vi "Node Status to gRPC Status.vi"(2 "Node Status":T1 {"Custom 8" format="%#_13g"}) -> (4 "gRPC Status":T4)   [LabVIEW 2021, in "CIFTemplateCommon.lvlib"]
uses:
  CIFTemplateCommon.lvlib
  CIFNodeCoreGrpc/CIFNodeCoreGrpc_server/RPC Messages/cif_nodecore_StatusData.ctl
  CIFNodeCoreGrpc/CIFNodeCoreGrpc_server/RPC Messages/cif_nodecore_StatusData_State.ctl
  CIFNodeCoreGrpc/CIFNodeCoreGrpc_server/RPC Messages/cif_nodecore_Error.ctl
  Typedef/Plugin Status.ctl
  Typedef/Plugin State.ctl
  Typedef/Simple Error.ctl
  CIFNodeCoreGrpc/CIFNodeCoreGrpc_server/CIFNodeCoreGrpc_server.lvlib
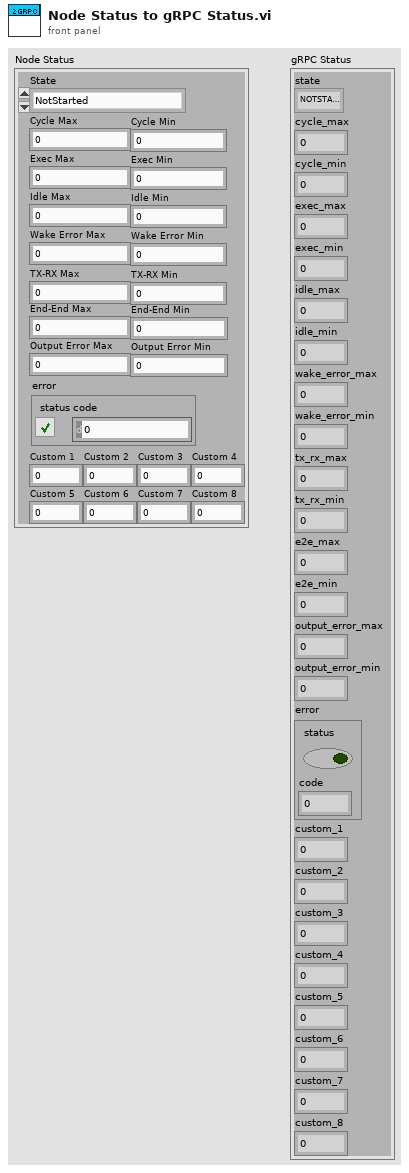
[diagram p1: front panel]
types:
  T1 = typedef "CIFTemplateCommon.lvlib/Plugin Status.ctl" = cluster{"State":T2, "Cycle Max":i32, "Cycle Min":i32, "Exec Max":i32, "Exec Min":i32, "Idle Max":i32, "Idle Min":i32, "Wake Error Max":i32, "Wake Error Min":i32, "TX-RX Max":i32, "TX-RX Min":i32, "End-End Max":i32, "End-End Min":i32, "Output Error Max":i32, "Output Error Min":i32, "error":T3, "Custom 1":u64, "Custom 2":u64, "Custom 3":u64, "Custom 4":u64, "Custom 5":dbl, "Custom 6":dbl, "Custom 7":dbl, "Custom 8":dbl}
  T2 = typedef "CIFTemplateCommon.lvlib/Plugin State.ctl" = enum32{"NotStarted", "Initialized", "Ready", "Running", "Shutdown"}
  T3 = typedef "CIFTemplateCommon.lvlib/Simple Error.ctl" = cluster{"status":bool, "code":i32}
  T4 = typedef "CIFNodeCoreGrpc_server.lvlib/cif_nodecore_StatusData.ctl" = cluster{"state":T5, "cycle_max":i32, "cycle_min":i32, "exec_max":i32, "exec_min":i32, "idle_max":i32, "idle_min":i32, "wake_error_max":i32, "wake_error_min":i32, "tx_rx_max":i32, "tx_rx_min":i32, "e2e_max":i32, "e2e_min":i32, "output_error_max":i32, "output_error_min":i32, "error":T6, "custom_1":u64, "custom_2":u64, "custom_3":u64, "custom_4":u64, "custom_5":dbl, "custom_6":dbl, "custom_7":dbl, "custom_8":dbl}
  T5 = typedef "CIFNodeCoreGrpc_server.lvlib/cif_nodecore_StatusData_State.ctl" = enum32{"NOTSTARTED", "INITIALIZED", "READY", "RUNNING", "SHUTDOWN"}
  T6 = typedef "CIFNodeCoreGrpc_server.lvlib/cif_nodecore_Error.ctl" = cluster{"status":bool, "code":i32}
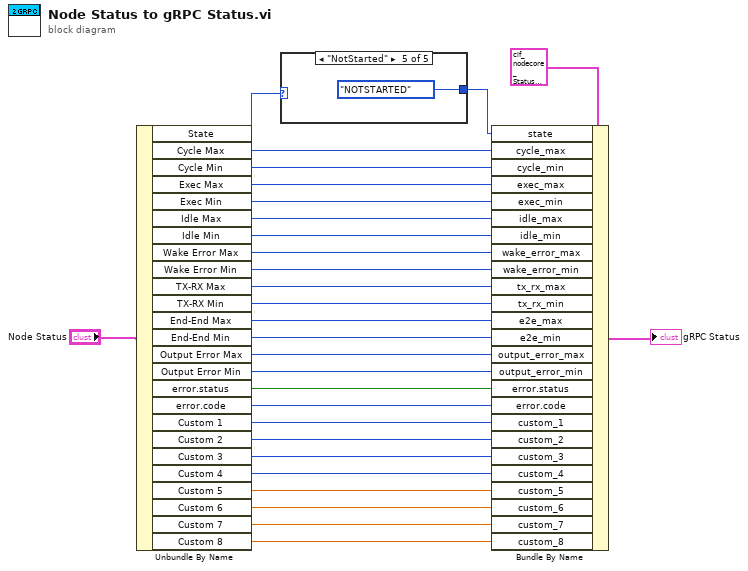
[diagram p0: block diagram]
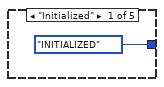
[diagram p2: hidden frame]
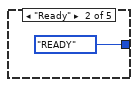
[diagram p3: hidden frame]
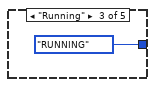
[diagram p4: hidden frame]
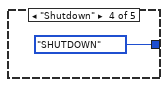
[diagram p5: hidden frame]
diagram:
  n1 = Unbundle By Name("Node Status") -> ("State"=w25:T2, "Cycle Max"=w24:i32, "Cycle Min"=w23:i32, "Exec Max"=w22:i32, "Exec Min"=w21:i32, "Idle Max"=w20:i32, "Idle Min"=w19:i32, "Wake Error Max"=w18:i32, "Wake Error Min"=w17:i32, "TX-RX Max"=w16:i32, "TX-RX Min"=w15:i32, "End-End Max"=w14:i32, "End-End Min"=w13:i32, "Output Error Max"=w12:i32, "Output Error Min"=w11:i32, "error.status"=w10:bool, "error.code"=w9:i32, "Custom 1"=w1:u64, "Custom 2"=w2:u64, "Custom 3"=w3:u64, "Custom 4"=w4:u64, "Custom 5"=w5:dbl, "Custom 6"=w6:dbl, "Custom 7"=w7:dbl, "Custom 8"=w8:dbl)
  n2 = case shown="\"NotStarted\"" w25 {
    tunnel: [cif_nodecore_StatusData_State."INITIALIZED" ("state") cif_nodecore_StatusData_State."READY" ("state") cif_nodecore_StatusData_State."RUNNING" ("state") cif_nodecore_StatusData_State."SHUTDOWN" ("state") cif_nodecore_StatusData_State."NOTSTARTED" ("state")] -> w26
    frame "Initialized" {
    }
    frame "Ready" {
    }
    frame "Running" {
    }
    frame "Shutdown" {
    }
    frame "NotStarted" {
    }
  }
  n3 = Bundle By Name(cluster=T4 {"state"=enum."NOTSTARTED", "cycle_max"=0, "cycle_min"=0, "exec_max"=0, "exec_min"=0, "idle_max"=0, "idle_min"=0, "wake_error_max"=0, "wake_error_min"=0, "tx_rx_max"=0, "tx_rx_min"=0, "e2e_max"=0, "e2e_min"=0, "output_error_max"=0, "output_error_min"=0, "error"={"status"=FALSE, "code"=0}, "custom_1"=0, "custom_2"=0, "custom_3"=0, "custom_4"=0, "custom_5"=0.0, "custom_6"=0.0, "custom_7"=0.0, "custom_8"=0.0} ("Message Data"), "state"=w26, "cycle_max"=w24, "cycle_min"=w23, "exec_max"=w22, "exec_min"=w21, "idle_max"=w20, "idle_min"=w19, "wake_error_max"=w18, "wake_error_min"=w17, "tx_rx_max"=w16, "tx_rx_min"=w15, "e2e_max"=w14, "e2e_min"=w13, "output_error_max"=w12, "output_error_min"=w11, "error.status"=w10, "error.code"=w9, "custom_1"=w1, "custom_2"=w2, "custom_3"=w3, "custom_4"=w4, "custom_5"=w5, "custom_6"=w6, "custom_7"=w7, "custom_8"=w8) -> (→"gRPC Status":T4)
